vi "z-wave-2.vi"(3 "index":i32, 5 "amplitutude":dbl=1.0) -> (0 "Waveform Graph 2":dbl[](graph)=[1.000817, 1.00105, 1.000103, 1.000151, 1.00033, 0.998936, 0.999535, 0.998932, 0.999805, 0.997953, 0.998416, 0.998677, 0.998281, 0.998354, 0.998007, 0.996458, 0.996038, 0.997315, 0.99629, 0.994986, 0.990277, 0.994125, 0.991847, 0.992764, 0.991279, 0.98921, 0.988805, 0.986694, 0.985855, 0.981276, 0.982225, 0.980965, 0.977334, 0.977021, 0.97472, 0.972876, 0.971043, 0.96981, 0.968379, 0.970814, 0.971608, 0.973723, 0.978493, 0.98633, 0.994463, 1.00176, 1.010046, 1.020141, 1.026156, 1.029629, 1.033377, 1.034634, 1.034348, 1.032787, 1.03134, 1.031697, 1.028913, 1.028134, 1.02646, 1.024693, 1.023765, 1.021838, 1.020238, 1.018643, 1.017274, 1.016255, 1.015458, 1.014319, 1.013925, 1.013988, 1.01085, 1.011457, 1.010237, 1.009642, 1.009866, 1.008764, 1.008303, 1.00851, 1.007199, 1.006652, 1.006823, 1.00616, 1.003738, 1.006106, 1.0063, 1.00483, 1.004944, 1.004568, 1.004054, 1.003758, 1.004019, 1.004157, 1.004165, 1.003884, 1.0038], 1 "element":dbl=1.000817, 2 "array size":i32=95)   [LabVIEW 2014]
panel:
  out "size(s)":i32=95
  in  "Waveform Graph":dbl[](graph)=[1.000817, 1.00105, 1.000103, 1.000151, 1.00033, 0.998936, 0.999535, 0.998932, 0.999805, 0.997953, 0.998416, 0.998677, 0.998281, 0.998354, 0.998007, 0.996458, 0.996038, 0.997315, 0.99629, 0.994986, 0.990277, 0.994125, 0.991847, 0.992764, 0.991279, 0.98921, 0.988805, 0.986694, 0.985855, 0.981276, 0.982225, 0.980965, 0.977334, 0.977021, 0.97472, 0.972876, 0.971043, 0.96981, 0.968379, 0.970814, 0.971608, 0.973723, 0.978493, 0.98633, 0.994463, 1.00176, 1.010046, 1.020141, 1.026156, 1.029629, 1.033377, 1.034634, 1.034348, 1.032787, 1.03134, 1.031697, 1.028913, 1.028134, 1.02646, 1.024693, 1.023765, 1.021838, 1.020238, 1.018643, 1.017274, 1.016255, 1.015458, 1.014319, 1.013925, 1.013988, 1.01085, 1.011457, 1.010237, 1.009642, 1.009866, 1.008764, 1.008303, 1.00851, 1.007199, 1.006652, 1.006823, 1.00616, 1.003738, 1.006106, 1.0063, 1.00483, 1.004944, 1.004568, 1.004054, 1.003758, 1.004019, 1.004157, 1.004165, 1.003884, 1.0038]
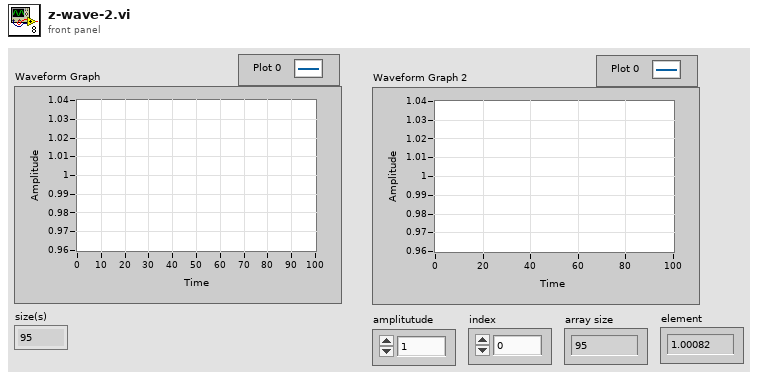
[diagram p1: front panel]
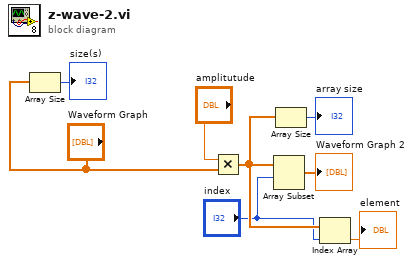
[diagram p0: block diagram]
diagram:
  n1 = Array Size(array="Waveform Graph") -> (size(s)=→"size(s)":i32)
  n2 = Multiply(x="amplitutude", y="Waveform Graph") -> (x*y=w4:dbl[])
  n3 = Array Subset(array=w4, index="index") -> (→"Waveform Graph 2":dbl[])  [unwired: 1 in]
  n4 = Array Size(array=w4) -> (size(s)=→"array size":i32)
  n5 = Index Array(array=w4, index="index") -> (element=→"element":dbl)
